vi "Control Main.vi"(10 "States":T1 format="%.4f", 11 "Target":T2={"Position"=0.0, "Invert"=TRUE} {"Position" min=-0.5 max=0.5 step=0.1 format="%.2g"}) -> (3 "PWM":dbl)   [LabVIEW 2018]
uses:
  Model/Target.ctl
  Model/States.ctl
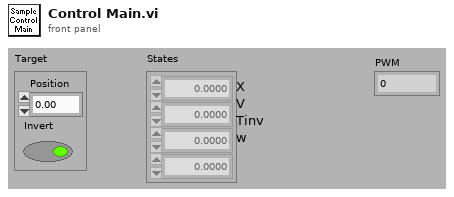
[diagram p1: front panel]
types:
  T1 = typedef "States.ctl" = dbl[]
  T2 = typedef "Target.ctl" = cluster{"Position":dbl, "Invert":bool}
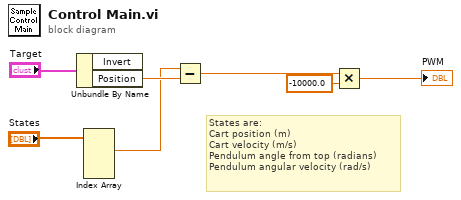
[diagram p0: block diagram]
diagram:
  # "States are:\nCart position (m)\nCart velocity (m/s)\nPendulum angle from top (radians)\nPendulum angular velocity (rad/s)"
  n1 = Unbundle By Name("Target") -> ("Position"=w6:dbl)  [unwired: 1 out]
  n2 = Index Array(array="States") -> (element #1=w3:dbl)  [unwired: 4 in, 3 out]
  n3 = Subtract(x=w3, y=w6) -> (x-y=w5:dbl)
  n4 = Multiply(x=w5, y=-10000.0 ("w")) -> (x*y=→"PWM":dbl)
